vi "ni579x Synchronize Signal.vi"(0 "sync.resources":T1, 1 "sync.cptr.FPGA I/O":refnum<k21>, 7 "enable":bool, 11 "edge":bool) -> (4 "sync.resources":T1, 10 "synchronization delay":u16, 15 "synchronized edge":bool)   [LabVIEW 2015, in "ni579x Synchronization v1 FPGA.lvlib"]
doc: "Synchronously realize a signal.\n\nIf this target is the master, it will distribute <B>edge</B> on the specified FPGA I/O line on the next falling edge of the CPTR (when <B>edge</B> is high). If this target is not the master, it will ignore <B>edge</B>. All targets (master or otherwise) will also read the FPGA I/O line. The <B>synchronized edge</B> output will go high on the next CPTR edge after the edge is read from the FPGA I/O line.\n\nNote: The input, <B>edge</B>, should be a pulse. This in enforced by the VI. There is a rising edge detector in the <B>edge</B> input. Also, after an edge is seen, another edge will not be recognized until after the edge distribution has completed. This means that the minimum time between edges for synchronization is one to two CPTR periods (it depends on when the edge is seen within the CPTR period).\n\n<B>Input Parameters</B>\n\n<B>sync.resources</B> identifies the Synchronization instance. 'sync.resources' is obtained from the ni579x Create VI of this library.\n\n<B>sync.cptr.FPGA I/O</B> is the FPGA I/O line that will be used to distribute/read the 'edge' for synchronization. This is commonly a PXI Trig line.\n\nNote: For large NI chassis, make sure the PXI Trig line is routed to all bus segments that have targets participating in synchronization.\n\n<B>enable</B> specifies whether to synchronize the input 'edge' or not.\n\nNote: If the 'sync.cptr.FPGA I/O' is a PXI Trig line, it will be floating until a target is specified as the master. 'enable' should be FALSE until after the host Synchronization VI executes to prevent erroneous outputs on 'synchronized edge'.\n\n<B>edge</B> is the input being synchronized. The very first block this input encounters is a rising edge detector, so the input signal, 'edge', will be treated as a pulse.\n\n<B>Output Parameters</B>\n\n<B>sync.resources</B> is the same instance that was passed in for 'sync.resources'.\n\n<B>synchronization delay</B> is the number of clock cycles of delay that were added by synchronizing the input 'edge'. This value is zero if 'enable' is false. If 'enable' is true, this value is only valid on the master target.\n\n<B>synchronized edge</B> is the synchronized input edge (if 'enable' is true).\n\nNote: If 'enable' is true, it's possible that 'synchronized edge' will be spuriously true BEFORE the host Synchronization VIs are run. It is recommended that 'enable' be held FALSE until after the host Synchronization VI executes."
uses:
  <instrlib>/ni579x/Synchronization/v1/FPGA/ni579x Synchronization v1 FPGA.lvlib
  <instrlib>/_niInstr/Basic Elements/v1/FPGA/niInstr Basic Elements v1 FPGA.lvlib
  <instrlib>/ni579x/Synchronization/v1/FPGA/Implementation/Resources.ctl
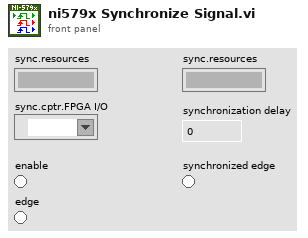
[diagram p1: front panel]
types:
  T1 = typedef "ni579x Synchronization v1 FPGA.lvlib/Resources.ctl" = cluster{"master":refnum<k21>, "meas.enable":refnum<k21>, "meas.ready":refnum<k21>, "meas.arm":refnum<k21>, "meas.valid":refnum<k21>, "meas.value":refnum<k21>, "meas.oversample clock":refnum<k21>, "meas.oversample factor":refnum<k21>, "cptr":refnum<k21>, "cptr.adjust":refnum<k21>, "cptr.period":refnum<k21>}
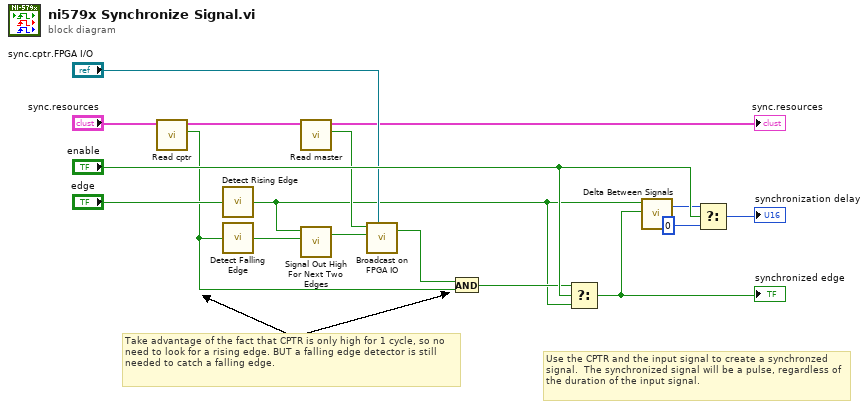
[diagram p0: block diagram]
diagram:
  # "Take advantage of the fact that CPTR is only high for 1 cycle, so no need to look for a rising edge. BUT a falling edge detector is still needed to catch a falling edge."
  # "Use the CPTR and the input signal to create a synchronzed signal.  The synchronized signal will be a pulse, regardless of the duration of the input signal."
  n1 = call <instrlib>:"Read cptr.vi"("sync.resources"="sync.resources") -> ("cptr"=w4:bool, "sync.resources"=w6:T1)  [unwired: 9 in]
  n2 = call <instrlib>:"Detect Rising Edge.vi"("signal"="edge") -> ("edge detected"=w1:bool)  [unwired: 14 in]
  n3 = call <instrlib>:"Detect Falling Edge.vi"("signal"=w4) -> ("edge detected"=w10:bool)  [unwired: 14 in]
  n4 = call <instrlib>:"Read master.vi"("sync.resources"=w6) -> ("master"=w5:bool, "sync.resources"=→"sync.resources":T1)  [unwired: 9 in]
  n5 = call <instrlib>:"Signal Out High For Next Two Edges.vi"("edge"=w10, "signal"=w1) -> ("signal for distribution"=w9:bool)  [unwired: 3 in]
  n6 = call <instrlib>:"Broadcast on FPGA IO.vi"("FPGA I/O"="sync.cptr.FPGA I/O", "signal in"=w9, "master"=w5) -> ("signal out"=w8:bool)  [unwired: 4 in]
  n7 = And(x=w8, y=w4) -> (x .and. y?=w12:bool)
  n8 = Select(t=w12, s="enable", f=w1) -> (s? t:f=w11:bool)
  "synchronized edge" <- w11
  n9 = call <instrlib>:"Delta Between Signals.vi"("second signal"=w11, "first signal"=w1) -> ("delta between signals"=w14:u16)  [unwired: 3 in]
  n10 = Select(t=w14, s="enable", f=u16 0) -> (s? t:f=→"synchronization delay":u16)
